vi "Main 9636.vi"() -> ()   [LabVIEW 2014]
uses:
  <vilib>/rvi/Emulation/niFpgaGetClockAttributes.vi
  <vilib>/rvi/Emulation/niFpgaSctlEmulationGetInTimedLoop.vi
  <vilib>/rvi/Emulation/niFpgaEmulationReportErrorSimple.vi
  <vilib>/rvi/eio/common/nirviEmuTemplateMethod_errors.vi
  <vilib>/rvi/Emulation/niFpgaCriticalErrorInLSC.vi
  <vilib>/eio/EIOMethodNode/EIOMethodNode.xnode
  <vilib>/eio/EIONode/EIONode.xnode
panel:
  out "error out":errorcluster
  out "Read DIO0":bool
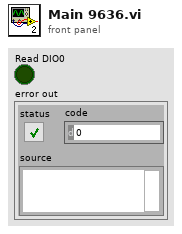
[diagram p1: front panel]
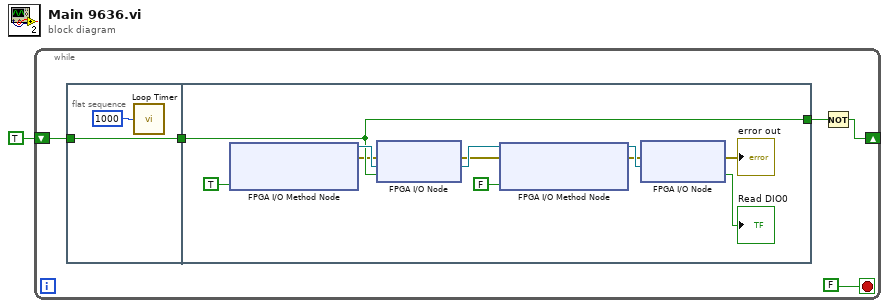
[diagram p0: block diagram]
diagram:
  n1 = while {
    shift-right: [w5] -> _
    shift-left: TRUE -> [w4]
    stop <- FALSE stop-if-true
    n2 = flat-sequence {
      tunnel: w4 -> [w7]
      tunnel: [w7] -> w3
      tunnel: w3 -> [w17]
      tunnel: [w17] -> w2
      frame #0 {
        n3 = call "Loop Timer"("Count(mSec)"=u16 1000) -> ()  [unwired: 1 out]
      }
      frame #1 {
        n4 = xnode "FPGA I/O Method Node"("Enable"=TRUE) -> ("error out"=w12:errorcluster, "FPGA I/O Out"=w18:refnum<k21>)  [unwired: 2 in]
        n5 = xnode "FPGA I/O Node"("error in"=w12, "I/O Item"=w17, "FPGA I/O In"=w18) -> ("error out"=w11:errorcluster, "FPGA I/O Out"=w16:refnum<k21>)
        n6 = xnode "FPGA I/O Method Node"("error in"=w11, "FPGA I/O In"=w16, "Enable"=FALSE) -> ("error out"=w10:errorcluster, "FPGA I/O Out"=w14:refnum<k21>)
        n7 = xnode "FPGA I/O Node"("error in"=w10, "FPGA I/O In"=w14) -> ("error out"=→"error out":errorcluster, "I/O Item"=→"Read DIO0":bool)  [unwired: 1 out]
      }
    }
    n8 = Not(x=w2) -> (.not. x?=w5:bool)
  }
